vi "Exercise1.20-Multi-Curve Display.vi"() -> ()   [LabVIEW 2013]
panel:
  out "XY Graph":cluster{dbl[], dbl[]}(graph)
  out "Waveform Graph":dynamicdata(graph)
  out "Waveform Graph":waveform(dbl)[](graph)
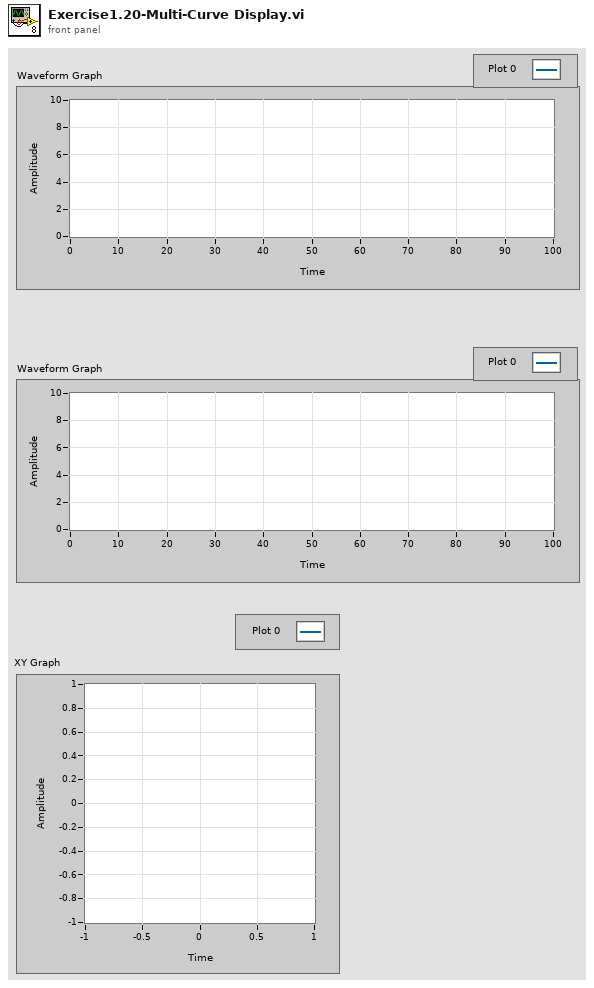
[diagram p1: front panel]
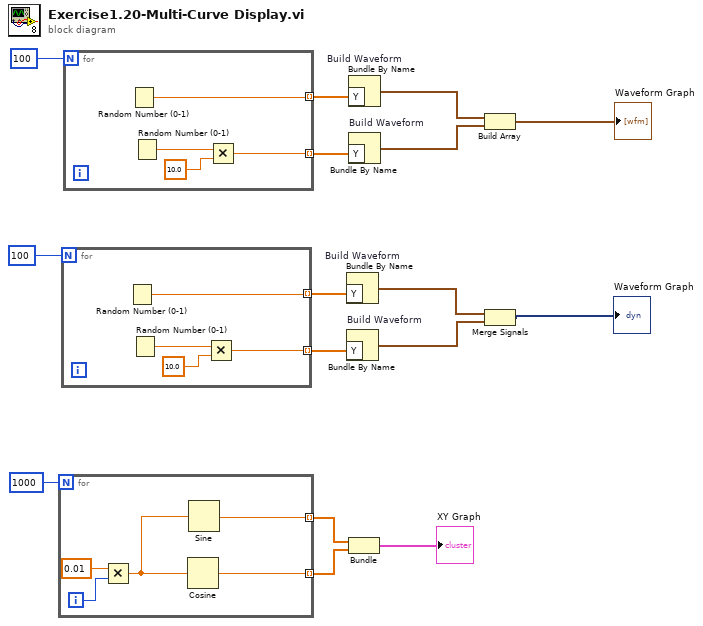
[diagram p0: block diagram]
diagram:
  n1 = for {
    N: 1000 -> [_]
    tunnel: [w21] -> w5 mode=indexing
    tunnel: [w17] -> w4 mode=indexing
    i -> [w20]
    n2 = Multiply(x=0.01, y=w20) -> (x*y=w18:dbl)
    n3 = Cosine(x=w18) -> (cos(x)=w17:dbl)
    n4 = Sine(x=w18) -> (sin(x)=w21:dbl)
  }
  n5 = for {
    N: 100 -> [_]
    tunnel: [w25] -> w10 mode=indexing
    tunnel: [w23] -> w9 mode=indexing
    n6 = Random Number (0-1)() -> (number: 0 to 1=w25:dbl)
    n7 = Random Number (0-1)() -> (number: 0 to 1=w24:dbl)
    n8 = Multiply(x=w24, y=10.0) -> (x*y=w23:dbl)
  }
  n9 = for {
    N: 100 -> [_]
    tunnel: [w29] -> w15 mode=indexing
    tunnel: [w27] -> w14 mode=indexing
    n10 = Random Number (0-1)() -> (number: 0 to 1=w29:dbl)
    n11 = Random Number (0-1)() -> (number: 0 to 1=w28:dbl)
    n12 = Multiply(x=w28, y=10.0) -> (x*y=w27:dbl)
  }
  n13 = Bundle By Name "Build Waveform"("Y"=w10) -> (w8:waveform(dbl))  [unwired: 1 in]
  n14 = Bundle By Name "Build Waveform"("Y"=w9) -> (w7:waveform(dbl))  [unwired: 1 in]
  n15 = Bundle By Name "Build Waveform"("Y"=w15) -> (w13:waveform(dbl))  [unwired: 1 in]
  n16 = Bundle By Name "Build Waveform"("Y"=w14) -> (w12:waveform(dbl))  [unwired: 1 in]
  n17 = Bundle "Bundle"(w5, w4) -> (→"XY Graph":cluster{dbl[], dbl[]})  [unwired: 1 in]
  n18 = Build Array "Build Array"(w13, w12) -> (→"Waveform Graph":waveform(dbl)[])
  n19 = Merge Signals "Merge Signals"(w8, w7) -> (→"Waveform Graph":dynamicdata)
